vi "log error.vi"(11 "String":string) -> (0 "error out":errorcluster)   [LabVIEW 2017]
uses:
  <vilib>/Utility/error.llb/DialogType.ctl
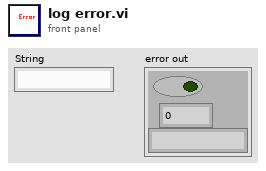
[diagram p1: front panel]
types:
  T1 = typedef "DialogType.ctl" = u16
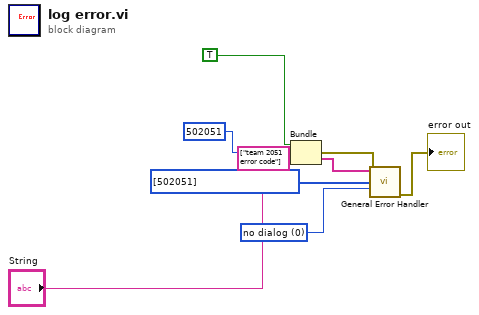
[diagram p0: block diagram]
diagram:
  w3 = T1 0 items=["no dialog", "OK message", "continue or stop message", "OK message + warnings", "continue/stop + warnings"] ("type of dialog (OK msg:1)")
  n1 = Bundle(TRUE, 502051, "String"="String") -> (w2:cluster{bool, i32, "String":string})  [unwired: 1 in]
  n2 = call <vilib>:"General Error Handler.vi"("[user-defined codes]"=i32[] [502051], "[user-defined descriptions]"=string[] ["team 2051 error code"], "type of dialog (OK msg:1)"=w3, "error in (no error)"=w2) -> ("error out"=→"error out":errorcluster)  [unwired: 7 in, 4 out]
